vi "Displayspeed_171213.vi"() -> (2 "DisplaySpeed":dbl, 3 "Waitin(ms)":dbl)   [LabVIEW 2016]
uses:
  Globaltracker.vi
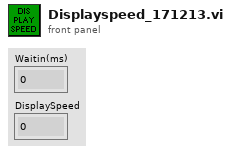
[diagram p1: front panel]
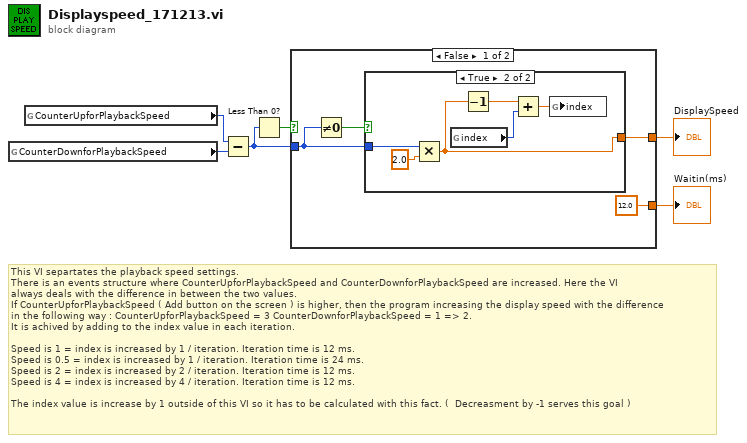
[diagram p0: block diagram]
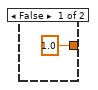
[diagram p2: hidden frame]
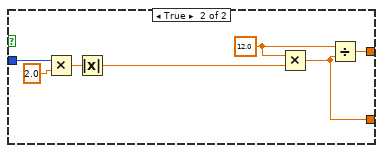
[diagram p3: hidden frame]
diagram:
  # "This VI separtates the playback speed settings. \nThere is an events structure where CounterUpforPlaybackSpeed and CounterDownforPlaybackSpeed are increased. Here the VI\nalways deals with the difference in between the two values. \nIf CounterUpforPlaybackSpeed ( Add button on the screen ) is higher, then the program increasing the display speed with the difference \nin the following way : CounterUpforPlaybackSpeed = 3 CounterDownforPlaybackSpeed = 1 => 2. \nIt is achived by adding to the index value in each iteration. \n\nSpeed is 1 = index is increased by 1 / iteration. Iteration time is 12 ms.\nSpeed is 0.5 = index is increased by 1 / iteration. Iteration time is 24 ms.\nSpeed is 2 = index is increased by 2 / iteration. Iteration time is 12 ms. \nSpeed is 4 = index is increased by 4 / iteration. Iteration time is 12 ms. \n\nThe index value is increase by 1 outside of this VI so it has to be calculated with this fact. (  Decreasment by -1 serves this goal )"
  n1 = global read "Globaltracker.vi" "CounterDownforPlaybackSpeed"() -> (w6:i16)
  n2 = global read "Globaltracker.vi" "CounterUpforPlaybackSpeed"() -> (w5:i16)
  n3 = Subtract(x=w5, y=w6) -> (x-y=w2:i16)
  n4 = Less Than 0?(x=w2) -> (x < 0?=w3:bool)
  n5 = case shown="False" w3 {
    tunnel: [12.0 w22] -> w4
    tunnel: w2 -> [w8 w21]
    tunnel: [w7 w18] -> w1
    frame False {
      n6 = Not Equal To 0?(x=w8) -> (x != 0?=w9:bool)
      n7 = case shown="True" w9 {
        tunnel: w8 -> [_ w16]
        tunnel: [1.0 ("_Speed_") w12] -> w7
        frame False {
        }
        frame True {
          n8 = Multiply(x=w16, y=2.0) -> (x*y=w12:dbl)
          n9 = global read "Globaltracker.vi" "index"() -> (w14:i16)
          n10 = Decrement(x=w12) -> (x-1=w15:dbl)
          n11 = Add(x=w15, y=w14) -> (x+y=w13:dbl)
          n12 = global write "Globaltracker.vi" "index"(w13) -> ()
        }
      }
    }
    frame True {
      w23 = 12.0 ("x")
      n13 = Multiply(x=w21, y=2.0) -> (x*y=w19:dbl)
      n14 = Absolute Value(x=w19) -> (abs(x)=w24:dbl)
      n15 = Multiply(x=w23, y=w24) -> (x*y=w22:dbl)
      n16 = Divide(x=w23, y=w22) -> (x/y=w18:dbl)
    }
  }
  "Waitin(ms)" <- w4
  "DisplaySpeed" <- w1
